vi "Comunicacion_Arcduino_buck.vi"() -> ()   [LabVIEW 2014]
panel:
  out "Waveform Chart":dynamicdata(graph)
  in  "Set Point":dbl(slide) scale=0.0..5.0
  in  "Kp 2":i32(knob) scale=0.0..1000.0
  in  "Kp 1":dbl(knob) scale=0.0..5.0
  in  "Ki":dbl(knob) scale=0.0..2000.0
  in  "Kd":dbl(knob) scale=0.0..2000.0
  in  "VISA resource name":refnum<visa-resource-name>
  in  "stop":bool
  in  "Velocidad de Conexion":enum16{"115200", "9600"}(ring)
  in  "error in (no error)":errorcluster
  # "Puerto de Com. Serial Elegido"
  # "Velocidad de Conexion"
  # "Punto de Consigna (V)"
  # "Control de Error de Entrada"
  # "Constante derivativa"
  # "Constante Integral"
  # "Constante Proporcional"
  # "Detener Ejecucion"
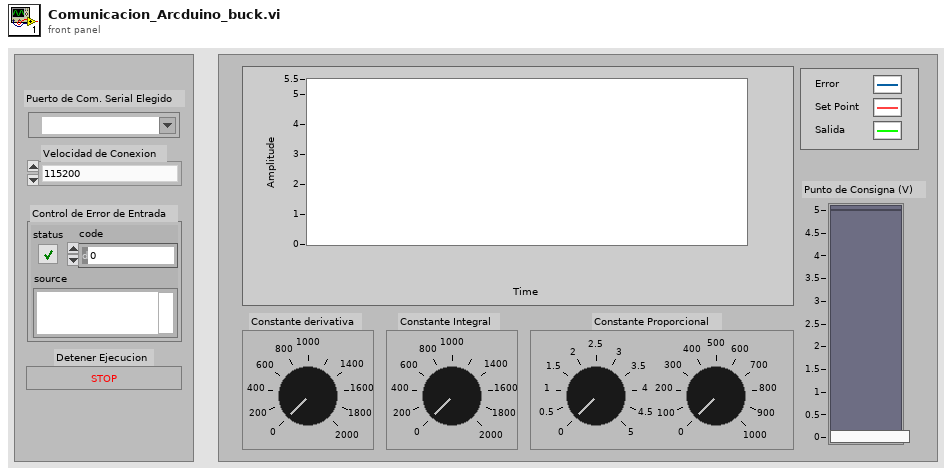
[diagram p1: front panel]
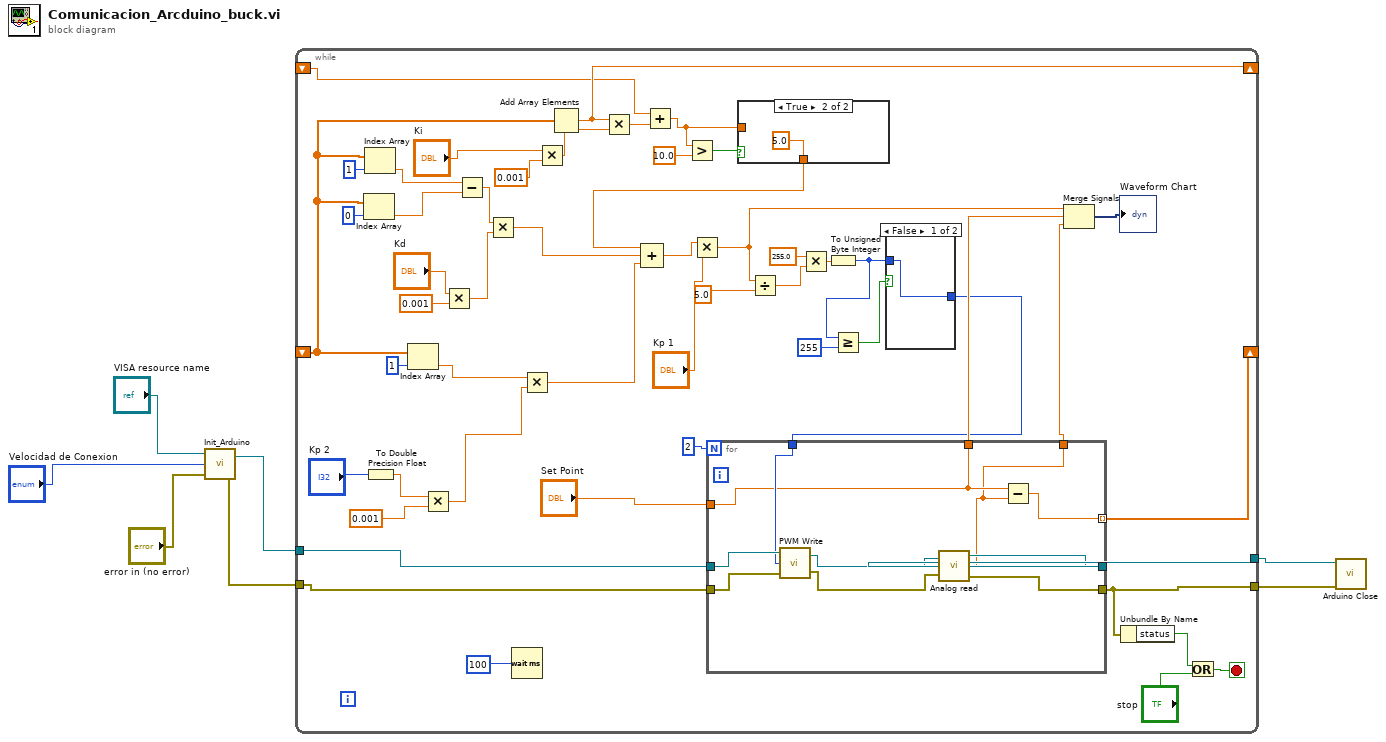
[diagram p0: block diagram]
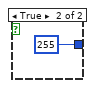
[diagram p3: hidden frame]
diagram:
  n1 = call "Init_Arduino.vi"("error in (no error)"="error in (no error)", "Velocidad de Conexion"="Velocidad de Conexion", "VISA Refnum in"="VISA resource name") -> ("error out"=w3:errorcluster, "VISA Refnum out"=w5:refnum<visa-resource-name>)
  n2 = while {
    tunnel: w3 -> [w58]
    tunnel: w5 -> [w59]
    tunnel: [w53] -> w1
    tunnel: [w54] -> w2
    shift-right: [w46] -> _
    shift-left: _ -> [w40]
    shift-right: [w12] -> _
    shift-left: _ -> [w9]
    stop <- w55 stop-if-true
    n3 = Index Array(array=w40, index=0) -> (element=w49:dbl)
    n4 = Index Array(array=w40, index=1) -> (element=w50:dbl)
    n5 = To Double Precision Float(number="Kp 2") -> (double precision float=w35:dbl)
    n6 = Index Array(array=w40, index=1) -> (element=w38:dbl)
    n7 = Multiply(x=w35, y=0.001) -> (x*y=w24:dbl)
    n8 = Multiply(x="Kd", y=0.001) -> (x*y=w44:dbl)
    n9 = Subtract(x=w50, y=w49) -> (x-y=w43:dbl)
    n10 = Multiply(x=w43, y=w44) -> (x*y=w34:dbl)
    n11 = Wait (ms)(milliseconds to wait=u32 100) -> ()  [unwired: 1 out]
    n12 = Multiply(x=w38, y=w24) -> (x*y=w33:dbl)
    n13 = Multiply(x="Ki", y=0.001) -> (x*y=w11:dbl)
    n14 = Add Array Elements(numeric array=w40) -> (sum=w12:dbl)
    n15 = Multiply(x=w12, y=w11) -> (x*y=w10:dbl)
    n16 = Add(x=w9, y=w10) -> (x+y=w8:dbl)
    n17 = Greater?(x=w8, y=10.0) -> (0:w16:bool)
    n18 = case shown="True" w16 {
      tunnel: w8 -> [w60 _]
      tunnel: [w60 5.0] -> w14
      frame False {
      }
      frame True {
      }
    }
    n19 = Compound Arithmetic op=ADD(w14, w34, w33) -> (w23:dbl)
    n20 = Multiply(x=w23, y="Kp 1") -> (x*y=w21:dbl)
    n21 = Divide(x=w21, y=5.0) -> (x/y=w30:dbl)
    n22 = Multiply(x=255.0, y=w30) -> (x*y=w28:dbl)
    n23 = To Unsigned Byte Integer(number=w28) -> (unsigned 8bit integer=w18:u8)
    n24 = Greater Or Equal?(x=w18, y=u8 255) -> (x >= y?=w19:bool)
    n25 = case shown="False" w19 {
      tunnel: w18 -> [w62 _]
      tunnel: [w62 u8 255] -> w17
      frame False {
      }
      frame True {
      }
    }
    n26 = for {
      N: 2 -> [_]
      tunnel: [w65] -> w46 mode=indexing
      tunnel: w59 -> [w73]
      tunnel: [w68] -> w53
      tunnel: w58 -> [w72]
      tunnel: [w69] -> w54
      tunnel: "Set Point" -> [w66]
      tunnel: w17 -> [w67]
      tunnel: [w66] -> w25
      tunnel: [w64] -> w26
      n27 = call "PWM Write.vi"("error in (no error)"=w72, "Ciclo de Trabajo"=w67, "VISA Refnum in"=w73) -> ("error out"=w70:errorcluster, "VISA Refnum out"=w71:refnum<visa-resource-name>)
      n28 = call "Analog read.vi"("VISA Refnum in"=w71, "error in (no error)"=w70) -> ("VISA Refnum out"=w68:refnum<visa-resource-name>, "Numeric"=w64:dbl, "error out"=w69:errorcluster)
      n29 = Subtract(x=w66, y=w64) -> (x-y=w65:dbl)
    }
    n30 = Merge Signals(w21, w25, w26) -> (→"Waveform Chart":dynamicdata)
    n31 = Unbundle By Name(w54) -> ("status"=w57:bool)
    n32 = Or(x=w57, y="stop") -> (x .or. y?=w55:bool)
  }
  n33 = call "Arduino Close.vi"("error in (no error)"=w2, "VISA Refnum in"=w1) -> ()  [unwired: 10 in]
